vi "硬件控制界面.vi"() -> ()   [LabVIEW 2013]
uses:
  <vilib>/DAQmx/create/channels.llb/DAQmx Create Channel (DO-Digital Output).vi
  <vilib>/DAQmx/create/channels.llb/DAQmx Create Channel (DI-Digital Input).vi
  GlobleVar/segment_size.vi
  <vilib>/DAQmx/read.llb/DAQmx Read (Digital Bool 1Line 1Point).vi
  <vilib>/DAQmx/write.llb/DAQmx Write (Digital 1D Bool 1Chan 1Samp).vi
panel:
  out "急停":bool
  out "触发":bool
  out "油压 2":dbl format="%0.1f"
  out "油压2":u8(slide) scale=0.0..20.0
  in  "电磁阀准备":bool
  out "油压 1":dbl format="%0.1f"
  out "行程 2":dbl format="%0.1f"
  out "行程":u8(slide) scale=0.0..20.0
  out "油压1":u8(slide) scale=0.0..20.0
  in  "开关":bool
  in  "L2":bool
  in  "L1":bool
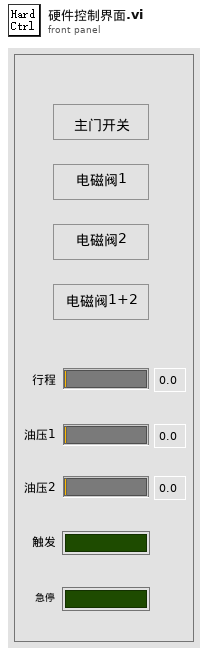
[diagram p1: front panel]
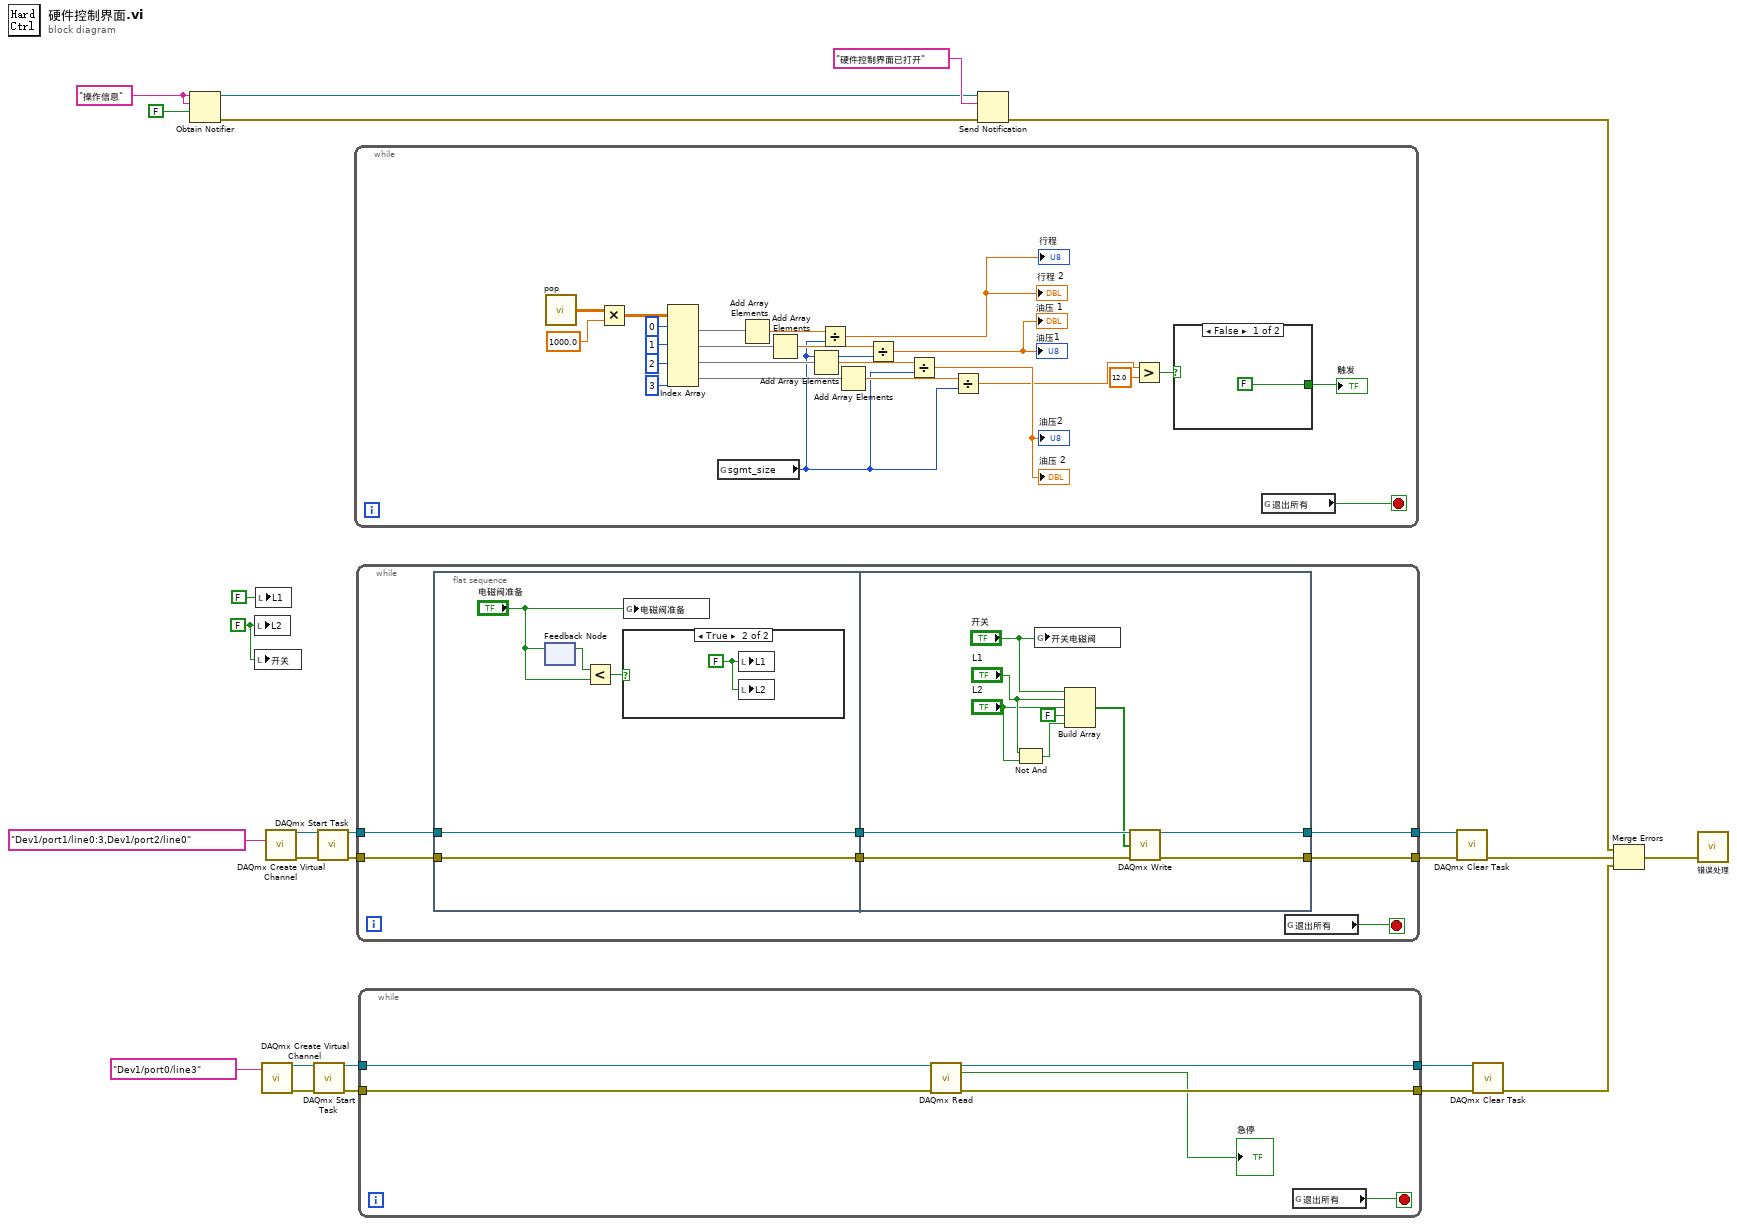
[diagram p0: block diagram]
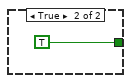
[diagram p3: hidden frame]
diagram:
  w10 = FALSE ("L2")
  w25 = "操作信息"
  n1 = Obtain Notifier(name (unnamed)=w25, notification data type=w25, create if not found? (T)=FALSE) -> (notifier out=w1:refnum<notifier>, error out=w22:errorcluster)  [unwired: 1 in, 1 out]
  n2 = local write "L2"(w10) -> ()
  n3 = local write "开关"(w10) -> ()
  n4 = local write "L1"(FALSE ("L1")) -> ()
  n5 = call-poly <vilib>:"DAQmx Create Virtual Channel.vi"("lines"=tag "Dev1/port0/line3") -> ("task out"=w9:refnum<k21>, "error out"=w8:errorcluster)  [unwired: 13 in]
  n6 = call-poly <vilib>:"DAQmx Create Virtual Channel.vi"("lines"=tag "Dev1/port1/line0:3,Dev1/port2/line0") -> ("task out"=w21:refnum<k21>, "error out"=w19:errorcluster)  [unwired: 13 in]
  n7 = call <vilib>:"DAQmx Start Task.vi"("task/channels in"=w9, "error in"=w8) -> ("task out"=w7:refnum<k21>, "error out"=w5:errorcluster)  [unwired: 12 in]
  n8 = call <vilib>:"DAQmx Start Task.vi"("task/channels in"=w21, "error in"=w19) -> ("task out"=w18:refnum<k21>, "error out"=w16:errorcluster)  [unwired: 12 in]
  n9 = while {
    stop <- w49 stop-if-true
    n10 = call "pop.vi"() -> ("Data out"=w45:dbl[][])  [unwired: 1 in]
    n11 = Multiply(x=w45, y=1000.0) -> (x*y=w46:dbl[][])
    n12 = Index Array(array=w46, index (row) #1=0 ("disabled index (col)"), index (row) #2=1 ("index (row)"), index (row) #3=2 ("index (row)"), index (row) #4=3 ("index (row)")) -> (element #1=w48:dbl[], element #2=w47:dbl[], element #3=w33:dbl[], element #4=w32:dbl[])  [unwired: 4 in]
    n13 = global read "segment_size.vi" "sgmt_size"() -> (w31:i32)
    n14 = Add Array Elements(numeric array=w48) -> (sum=w43:dbl)
    n15 = Add Array Elements(numeric array=w47) -> (sum=w41:dbl)
    n16 = Add Array Elements(numeric array=w33) -> (sum=w35:dbl)
    n17 = Divide(x=w43, y=w31) -> (x/y=→"行程 2" →"行程":dbl)
    n18 = Add Array Elements(numeric array=w32) -> (sum=w34:dbl)
    n19 = Divide(x=w41, y=w31) -> (x/y=→"油压 1" →"油压1":dbl)
    n20 = Divide(x=w35, y=w31) -> (x/y=→"油压2" →"油压 2":dbl)
    n21 = Divide(x=w34, y=w31) -> (x/y=w26:dbl)
    n22 = Greater?(x=w26, y=12.0) -> (0:w30:bool)
    n23 = case shown="False" w30 {
      tunnel: [FALSE TRUE ("电气")] -> w28
      frame False {
      }
      frame True {
      }
    }
    "触发" <- w28
    n24 = global read "退出所有.vi" "退出所有"() -> (w49:bool)
  }
  n25 = while {
    tunnel: w18 -> [w56]
    tunnel: [w55] -> w17
    tunnel: w16 -> [w53]
    tunnel: [w52] -> w15
    stop <- w58 stop-if-true
    n26 = flat-sequence {
      tunnel: [w60] -> w57
      tunnel: w56 -> [w60]
      tunnel: [w59] -> w54
      tunnel: w53 -> [w59]
      tunnel: w57 -> [w74]
      tunnel: [w73] -> w55
      tunnel: w54 -> [w72]
      tunnel: [w71] -> w52
      frame #0 {
        n27 = feedback #1() -> (w62:bool)  [unwired: 1 in]
        n28 = feedback-in #1("电磁阀准备") -> ()
        n29 = Less?(x=w62, y="电磁阀准备") -> (x < y?=w63:bool)
        n30 = case shown="True" w63 {
          frame False {
          }
          frame True {
            w64 = FALSE
            n31 = local write "L1"(w64) -> ()
            n32 = local write "L2"(w64) -> ()
          }
        }
        n33 = global write "电磁阀准备.vi" "电磁阀准备"("电磁阀准备") -> ()
      }
      frame #1 {
        n34 = Not And(1:"L2", 2:"L1") -> (0:w66:bool)
        n35 = global write "开关电磁阀.vi" "开关电磁阀"("开关") -> ()
        n36 = Build Array("开关", "L1", "L2", FALSE ("element"), w66) -> (w70:bool[])
        n37 = call-poly <vilib>:"DAQmx Write.vi"("task/channels in"=w74, "data"=w70, "error in"=w72) -> ("task out"=w73:refnum<k21>, "error out"=w71:errorcluster)  [unwired: 10 in, 1 out]
      }
    }
    n38 = global read "退出所有.vi" "退出所有"() -> (w58:bool)
  }
  n39 = while {
    tunnel: w7 -> [w79]
    tunnel: [w78] -> w6
    tunnel: w5 -> [w77]
    tunnel: [w76] -> w4
    stop <- w80 stop-if-true
    n40 = call-poly <vilib>:"DAQmx Read.vi"("task/channels in"=w79, "error in"=w77) -> ("task out"=w78:refnum<k21>, "data"=→"急停":bool, "error out"=w76:errorcluster)  [unwired: 11 in]
    n41 = global read "退出所有.vi" "退出所有"() -> (w80:bool)
  }
  n42 = Send Notification(notification="硬件控制界面已打开", notifier=w1, error in (no error)=w22) -> (error out=w12:errorcluster)  [unwired: 1 out]
  n43 = call <vilib>:"DAQmx Clear Task.vi"("task in"=w17, "error in"=w15) -> ("error out"=w14:errorcluster)  [unwired: 13 in]
  n44 = call <vilib>:"DAQmx Clear Task.vi"("task in"=w6, "error in"=w4) -> ("error out"=w3:errorcluster)  [unwired: 13 in]
  n45 = Merge Errors(w12, w14, w3) -> (w13:errorcluster)
  n46 = call "错误处理.vi"("error in (no error)"=w13) -> ()  [unwired: 2 in]
